vi "create PlayerCell.vi"(8 "error in (no error)":errorcluster, 10 "Player":refnum<class "Player.lvclass">, 11 "PlayerCell in":refnum<class "PlayerCell.lvclass">) -> (0 "error out":errorcluster, 3 "PlayerCell out":refnum<class "PlayerCell.lvclass">)   [LabVIEW 2019, in "PlayerCell.lvclass"]
uses:
  PlayerCell.lvclass
  Player/Player.lvclass
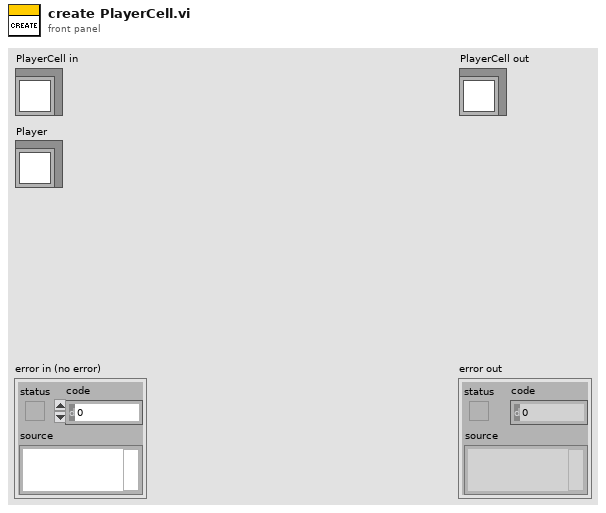
[diagram p1: front panel]
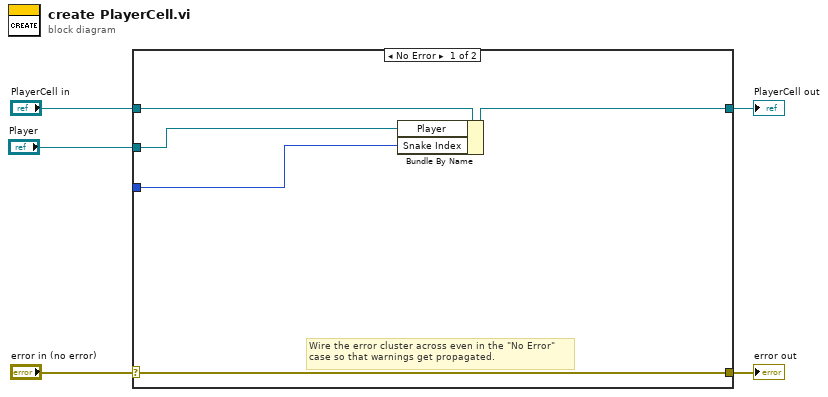
[diagram p0: block diagram]
diagram:
  n1 = case shown="No Error" "error in (no error)" {
    selector: "error in (no error)" -> [w10 w13]
    tunnel: [w10 w13] -> w5
    tunnel: [w9 w12] -> w3
    tunnel: "PlayerCell in" -> [w11 w12]
    tunnel: "Player" -> [w8 _]
    tunnel: [w7 _] -> w1
    frame No Error {
      # "Wire the error cluster across even in the \"No Error\"\ncase so that warnings get propagated."
      n2 = Bundle By Name(cluster=w11, "Player"=w8, "Snake Index"=w7) -> (w9:refnum<class "PlayerCell.lvclass">)
    }
    frame Error {
    }
  }
  "error out" <- w5
  "PlayerCell out" <- w3
